vi "Global1.vi"() -> ()   [LabVIEW 2020]
panel:
  in  "SQL":string
  in  "工位追溯码":string
  in  "USER_ID":string
  in  "DEVICE_ID":string
  in  "CODE_ID":string
  in  "前序DEVICE_ID":string
  in  "PRODUCT_ID":string
  in  "DEVICE_PC_ID":string
  in  "传感器码":string
  out "生产结果":string
  out "电机工位生产结果":string
  in  "联机模式":enum16{"单机", "联网"}(ring)=enum."联网"
  out "用户信息":T1
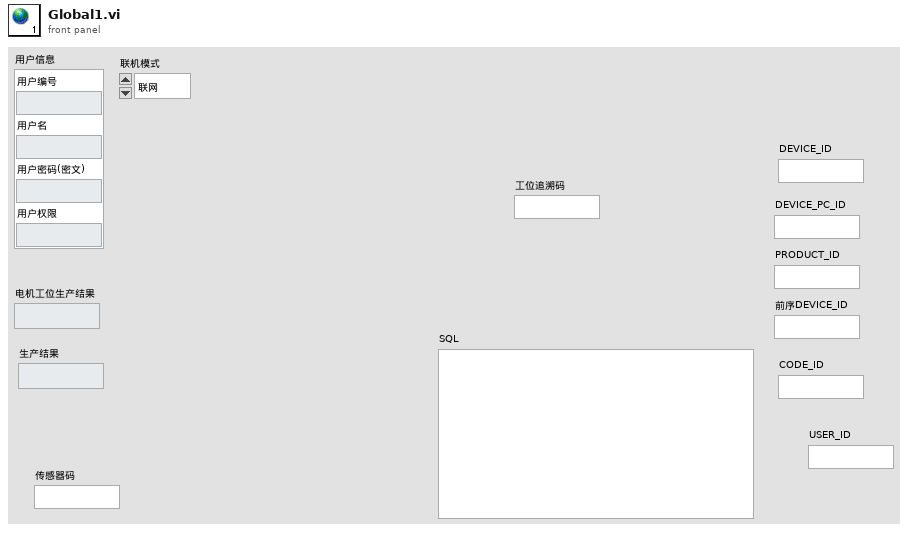
[diagram p1: front panel]
types:
  T1 = cluster{"用户编号":string, "用户名":string, "用户密码(密文)":string, "用户权限":string}
diagram:
